vi "Graph-Multi.vi"() -> ()   [LabVIEW 2020]
doc: "Illustrates the various single plot and multi plot data types that the waveform graph accepts. \n\nUse the waveform graph to display data that is uniformly distributed along the X-axis. This is particularly useful when displaying data that was sampled at a uniform rate. See XY Graph.vi for examples of how to use the XY graph."
panel:
  out "MultiGraph3":cluster{"x0":i32, "dx":i32, dbl[]}[](graph)
  out "MultiGraph2":cluster{dbl[]}[](graph)
  out "MultiGraph1":dbl[][](graph)
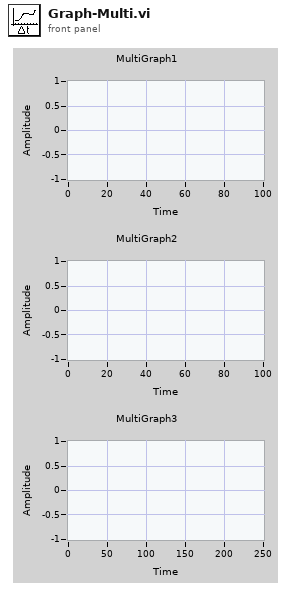
[diagram p1: front panel]
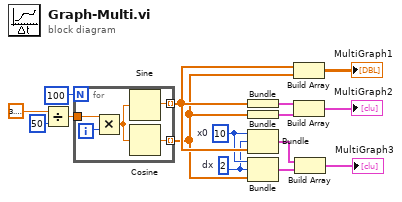
[diagram p0: block diagram]
diagram:
  w1 = 2  # dx
  w2 = 10  # x0
  n1 = Divide(x=3.141592653589793, y=50) -> (x/y=w13:dbl)
  n2 = for {
    N: 100 -> [_]
    tunnel: w13 -> [w20]
    tunnel: [w17] -> w10 mode=indexing
    tunnel: [w16] -> w9 mode=indexing
    i -> [w19]
    n3 = Multiply(x=w20, y=w19) -> (x*y=w18:dbl)
    n4 = Sine(x=w18) -> (sin(x)=w17:dbl)
    n5 = Cosine(x=w18) -> (cos(x)=w16:dbl)
  }
  n6 = Bundle "Bundle"(w10) -> (w11:cluster{dbl[]})  [unwired: 1 in]
  n7 = Bundle(w9) -> (w12:cluster{dbl[]})  [unwired: 1 in]
  n8 = Bundle("x0"=w2, "dx"=w1, w10) -> (w7:cluster{"x0":i32, "dx":i32, dbl[]})  [unwired: 1 out]
  n9 = Bundle("x0"=w2, "dx"=w1, w9) -> (w8:cluster{"x0":i32, "dx":i32, dbl[]})  [unwired: 1 out]
  n10 = Build Array "Build Array"(w10, w9) -> (→"MultiGraph1":dbl[][])
  n11 = Build Array(w11, w12) -> (→"MultiGraph2":cluster{dbl[]}[])
  n12 = Build Array(w7, w8) -> (→"MultiGraph3":cluster{"x0":i32, "dx":i32, dbl[]}[])
